vi "checkInputAndBroadcast.vi"(8 "error in (no error)":errorcluster, 10 "inputString":string, 11 "TcpServerBase in":refnum<class "TcpServerBase.lvclass">) -> (0 "error out":errorcluster, 3 "TcpServerBase out":refnum<class "TcpServerBase.lvclass">)   [LabVIEW 2018, in "TcpServerBase.lvclass"]
doc: "Check the input string: If is not empty, the input is an unknown message and is sent as a GenRead user event to the user. If is empty, nothing is done in this VI, and the GenRead user event is used to let the user know about the connection status of TCP clients."
uses:
  TcpServerBase.lvclass
  typedef/connStatusCluster.ctl
  TcpServerBase.lvclass/TcpServerBase.ctl
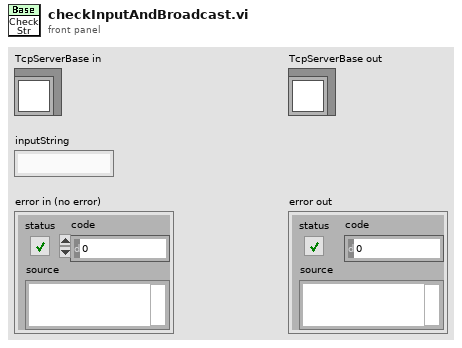
[diagram p1: front panel]
types:
  T1 = typedef "TcpServerBase.lvclass/connStatusCluster.ctl" = cluster{"connStatus":bool, "message":string}
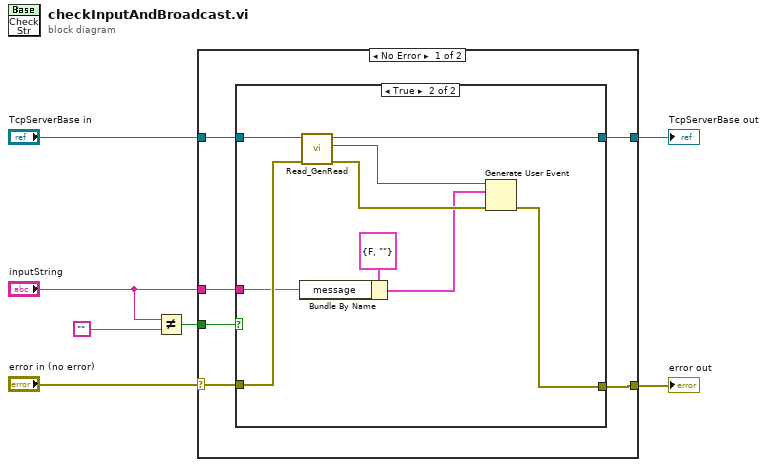
[diagram p0: block diagram]
diagram:
  n1 = Not Equal?(x="inputString", y="") -> (x != y?=w3:bool)
  n2 = case shown="No Error" "error in (no error)" {
    selector: "error in (no error)" -> [w13 w25]
    tunnel: [w12 w26] -> w6
    tunnel: "TcpServerBase in" -> [w11 w26]
    tunnel: [w10 w25] -> w4
    tunnel: w3 -> [w9 _]
    tunnel: "inputString" -> [w8 _]
    frame No Error {
      n3 = case shown="True" w9 {
        tunnel: w13 -> [w15 w22]
        tunnel: [w14 w21] -> w12
        tunnel: w11 -> [w14 w20]
        tunnel: [w15 w19] -> w10
        tunnel: w8 -> [_ w16]
        frame False {
        }
        frame True {
          n4 = Bundle By Name(cluster=T1 {"connStatus"=FALSE, "message"=""} ("event data"), "message"=w16) -> (w18:T1)
          n5 = call "Read_GenRead.vi"("error in (no error)"=w22, "TcpServerBase in"=w20) -> ("error out"=w23:errorcluster, "GenRead"=w24:refnum<user-event>, "TcpServerBase out"=w21:refnum<class "TcpServerBase.lvclass">)  [unwired: 7 in]
          n6 = Generate User Event(user event=w24, event data cluster=w18, error in=w23) -> (error out=w19:errorcluster)  [unwired: 1 in, 1 out]
        }
      }
    }
    frame Error {
    }
  }
  "TcpServerBase out" <- w6
  "error out" <- w4
